vi "Digital Open_XX.vi"(8 "Error In":errorcluster, 11 "LINX Resource":T3) -> (0 "Error Out":errorcluster, 3 "LINX Resource":T3)   [LabVIEW 2011, in "LVH-LINX.lvlib"]
uses:
  LVH-LINX.lvlib
  Private/Type Defs/LINX Ref.ctl
  Private/Type Defs/Platform.ctl
  Private/Type Defs/Interface.ctl
  Private/Type Defs/TCP Config.ctl
  Private/Type Defs/LINX Device Config.ctl
  Private/Type Defs/Peripherals/Digital/Digital Pin Configuration.ctl
  Private/Type Defs/Peripherals/Digital/Digital Pin Mode.ctl
  Private/myRIO/myLINX.lvlib
  Private/Device/Device.lvlib
panel:
  in  "Pins":T1[](array[typedef])
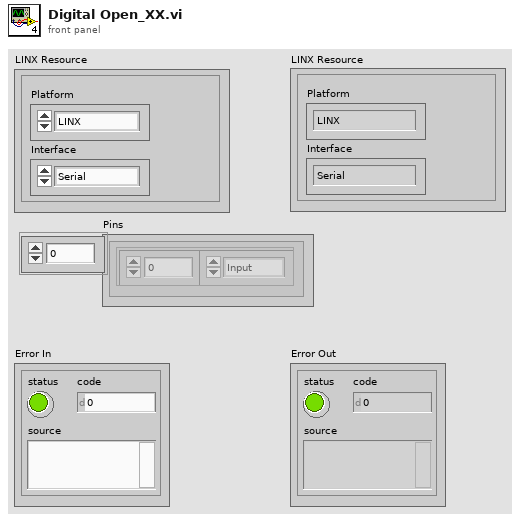
[diagram p1: front panel]
types:
  T1 = typedef "LVH-LINX.lvlib/Digital Pin Configuration.ctl" = cluster{"Pin Number":u8, "Digital Pin Mode":T2}
  T2 = typedef "LVH-LINX.lvlib/Digital Pin Mode.ctl" = enum8{"Input", "Output"}
  T3 = typedef "LVH-LINX.lvlib/LINX Ref.ctl" = cluster{"Platform":T4, "Interface":T5, "TCP Configuration":T6, "COM Port":refnum<visa-resource-name>, "LINX Device Config":T7}
  T4 = typedef "LVH-LINX.lvlib/Platform.ctl" = enum16{"LINX", "myRIO"}
  T5 = typedef "LVH-LINX.lvlib/Interface.ctl" = enum16{"Serial", "TCP"}
  T6 = typedef "LVH-LINX.lvlib/TCP Config.ctl" = cluster{"IP Address":string, "Port":dbl}
  T7 = typedef "LVH-LINX.lvlib/LINX Device Config.ctl" = cluster{"Interface":T5, "COM Port":refnum<visa-resource-name>, "Packet Number":u16, "TCP Configuration":T6, "Device Family":u8, "Device ID":u8, "Device Name":string}
  T8 = typedef "DIO.lvlib/DIO Reference.ctl" = cluster{"myRIO Reference":T9, "DIO Channels List":T13}
  T9 = typedef "myRIO Generic Hardware Reference.ctl" = cluster{"myRIO Model":T10, "myRIO Hardware Reference":T11}
  T10 = typedef "Hardware Version Enum.ctl" = enum16{"Unknown", "myRIO-1900", "myRIO-1950"}
  T11 = typedef "myRIO v1.0 Reference.ctl" = cluster{"Generic FPGA Reference":T12, "Allow multiple opens":bool}
  T12 = typedef "Generic FPGA Reference.ctl" = refnum<k20>
  T13 = typedef "DIO Channels List.ctl" = T14[]
  T14 = typedef "DIO Channels Enum.ctl" = enum16{"Not Connected", "C/DIO0", "C/DIO1", "C/DIO2", "C/DIO3", "C/DIO4", "C/DIO5", "C/DIO6", "C/DIO7", "A/DIO0", "A/DIO1", "A/DIO2", "A/DIO3", "A/DIO4", "A/DIO5", "A/DIO6", "A/DIO7", "A/DIO8", "A/DIO9", "A/DIO10", "A/DIO11", "A/DIO12", "A/DIO13", "A/DIO14", "A/DIO15", "B/DIO0", "B/DIO1", "B/DIO2", "B/DIO3", "B/DIO4", "B/DIO5", "B/DIO6", "B/DIO7", "B/DIO8", "B/DIO9", "B/DIO10", "B/DIO11", "B/DIO12", "B/DIO13", "B/DIO14", "B/DIO15", "LED0", "LED1", "LED2", "LED3", "Button0"}
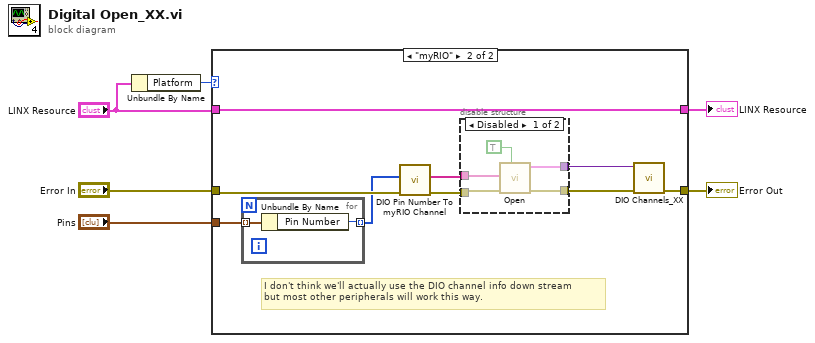
[diagram p0: block diagram]
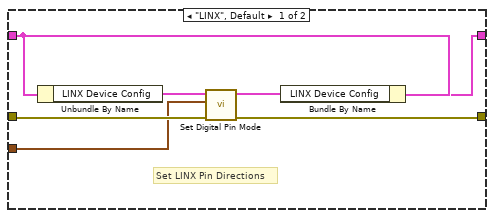
[diagram p2: hidden frame]
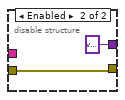
[diagram p3: hidden frame]
diagram:
  n1 = Unbundle By Name("LINX Resource") -> ("Platform"=w6:T4)
  n2 = case shown="\"myRIO\"" w6 {
    tunnel: "Error In" -> [w13 w21]
    tunnel: "LINX Resource" -> [w9 w22]
    tunnel: [w12 w17] -> w3
    tunnel: [w8 w22] -> w2
    tunnel: "Pins" -> [w10 w15]
    frame "LINX", Default {
      # "Set LINX Pin Directions"
      n3 = Unbundle By Name(w9) -> ("LINX Device Config"=w11:T7)
      n4 = call "Set Digital Pin Mode.vi"("Error In"=w13, "Digtal Pin Modes"=w10, "LINX Device Config"=w11) -> ("Error Out"=w12:errorcluster, "LINX Device Config"=w7:T7)  [unwired: 7 in]
      n5 = Bundle By Name(cluster=w9, "LINX Device Config"=w7) -> (w8:T3)
    }
    frame "myRIO" {
      # "I don't think we'll actually use the DIO channel info down stream\nbut most other peripherals will work this way."
      n6 = for {
        tunnel: w15 -> [w24] mode=indexing
        tunnel: [w23] -> w14 mode=indexing
        n7 = Unbundle By Name(w24) -> ("Pin Number"=w23:u8)
      }
      n8 = call "DIO Pin Number To myRIO Channel.vi"("Error In"=w21, "DIO Pins"=w14) -> ("Error Out"=w19:errorcluster, "DIO Channels"=w20:string[])  [unwired: 8 in]
      n9 = disable-structure shown="Disabled" {
        disable-tunnel: w20 -> [w29 _]
        disable-tunnel: w19 -> [w28 w31]
        disable-tunnel: [w27 w31] -> w18
        disable-tunnel: [w25 variant ("DIO Channel")] -> w16
        frame Disabled {
          n10 = call <vilib>:"Open.vi"("Allow multiple opens?"=TRUE, "error in (no error)"=w28, "Channel Names"=w29) -> ("error out"=w27:errorcluster, "DIO Ref Out"=w25:T8)  [unwired: 7 in]
        }
        frame Enabled {
        }
      }
      n11 = call "DIO Channels_XX.vi"("Error In"=w18, "DIO Channel"=w16) -> ("Error Out"=w17:errorcluster)  [unwired: 8 in, 1 out]
    }
  }
  "Error Out" <- w3
  "LINX Resource" <- w2
